vi "Save As Measurement Service template [Adv UI].vi"(8 "error in":errorcluster, 10 "measurement service name":string, 11 "project ref":refnum<vi>) -> (0 "error out":errorcluster)   [LabVIEW 2020, in "MeasurementService Editor.lvlib"]
uses:
  MeasurementService Editor.lvlib
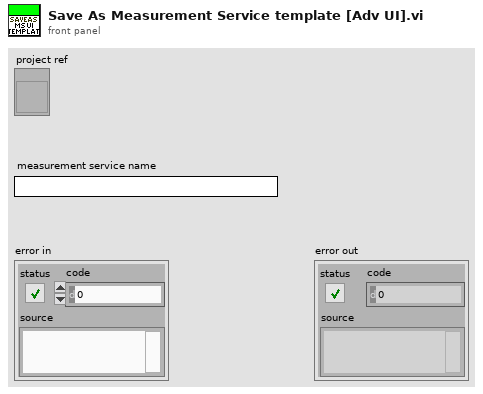
[diagram p1: front panel]
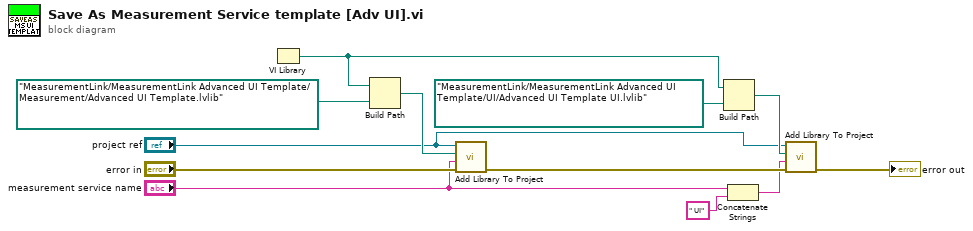
[diagram p0: block diagram]
diagram:
  n1 = VI Library() -> (path=w7:path)
  n2 = Build Path(base path=w7, name or relative path=path "MeasurementLink/MeasurementLink Advanced UI Template/Measurement/Advanced UI Template.lvlib" ("Library Path")) -> (appended path=w10:path)
  n3 = call "Add Library To Project.vi"("error in"="error in", "new library name"="measurement service name", "library path"=w10, "project ref"="project ref") -> ("error out"=w9:errorcluster)  [unwired: 7 in]
  n4 = Build Path(base path=w7, name or relative path=path "MeasurementLink/MeasurementLink Advanced UI Template/UI/Advanced UI Template UI.lvlib" ("Library Path")) -> (appended path=w6:path)
  n5 = Concatenate Strings("measurement service name", " UI" ("string")) -> (w3:string)
  n6 = call "Add Library To Project.vi"("error in"=w9, "new library name"=w3, "library path"=w6, "project ref"="project ref") -> ("error out"=→"error out":errorcluster)  [unwired: 7 in]
